vi "FestoCPX.Valve(2out2in).WithStop.vi"(4 "Delay [ms] (0)":u32, 6 "Timeout [ms] (5000)":u32=5000, 8 "error in (no error)":errorcluster, 9 "Position":T3, 10 "Valve outputs":T1[](array[typedef]), 11 "Inputs":T2[](array[typedef])) -> (0 "error out":errorcluster, 3 "Timeout?":bool)   [LabVIEW 2016]
uses:
  FestoCPX.DI.Data.States.Get.vi
  FestoCPX.DO.Data.States.Clear.vi
  FestoCPX.DI.Data.State.Get.vi
  Station/Station.ValvePosition.ctl
  FestoCPX.DI.Signal.ctl
  FestoCPX.DO.Signal.ctl
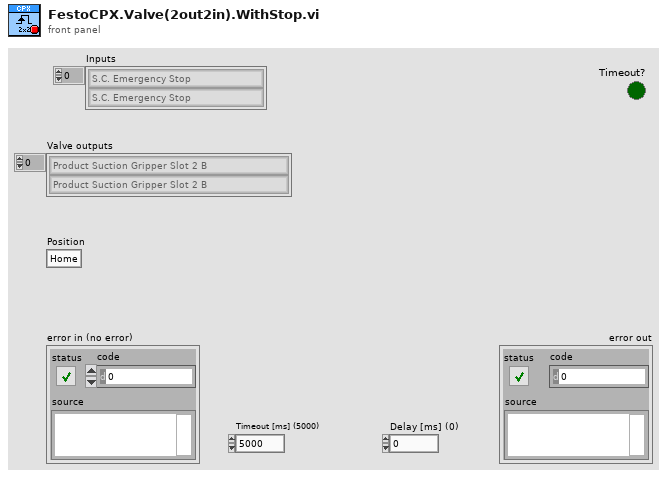
[diagram p1: front panel]
types:
  T1 = typedef "FestoCPX.DO.Signal.ctl" = enum16{"Safety Reset", "Air Main Valve", "Door Lock", "Button LED Start", "Button LED Stop", "Button LED Control", "Traffic LED Red", "Traffic LED Orange", "Traffic LED Green", "Horn", "Laser Interlock", "Laser Trigger", "Laser Fume Extractor", "Product Suction Gripper Slot 1 A", "Product Suction Gripper Slot 1 B", "Product Suction Gripper Slot 2 A", "Product Suction Gripper Slot 2 B", "Product Suction Gripper Slot 3 A", "Product Suction Gripper Slot 3 B", "Product Suction Gripper Slot 4 A", "Product Suction Gripper Slot 4 B", "Product Suction Gripper Final A", "Product Suction Gripper Final B", "Lamp", "Q1 Product Move Work", "Q1 Product Move Home", "Q2 Table Turn Work", "Q2 Table Turn Home", "Q3 Product Lift A", "Q3 Product Lift B", "Q4 Product Arm OK", "Q4 Product Arm NOK", "Q5 Product Arm Work", "Q6 Product BlowOut A", "Q6 Product BlowOut B"}
  T2 = typedef "FestoCPX.DI.Signal.ctl" = enum16{"S.C. Emergency Stop", "S.C. Side Door Close", "S.C. Front Door Close", "S.C. Front Door Secured", "Button Start", "Button Stop", "Button Control", "Product Move Home", "Product Move Work", "Table Position", "Table Lock", "Product Lift A Home", "Product Lift B Home", "Product Arm OK", "Product Arm NOK", "Product Arm Work", "Revolver ID 1", "Revolver ID 2", "Revolver ID 3", "Revolver ID 4", "Revolver ID 5", "Air Pressure Inside", "Air Pressure Inlet", "Product Slot 1 A Present", "Product Slot 1 B Present", "Product Slot 2 A Present", "Product Slot 2 B Present", "Product Slot 3 A Present", "Product Slot 3 B Present", "Product Slot 4 A Present", "Product Slot 4 B Present", "Product Final A Present", "Product Final B Present", "Product Output A Present", "Product Output B Present", "Product Container OK Present", "Product Container NOK Present", "Fork ID 1", "Fork ID 2"}
  T3 = typedef "Station.ValvePosition.ctl" = enum16{"Home", "Work"}
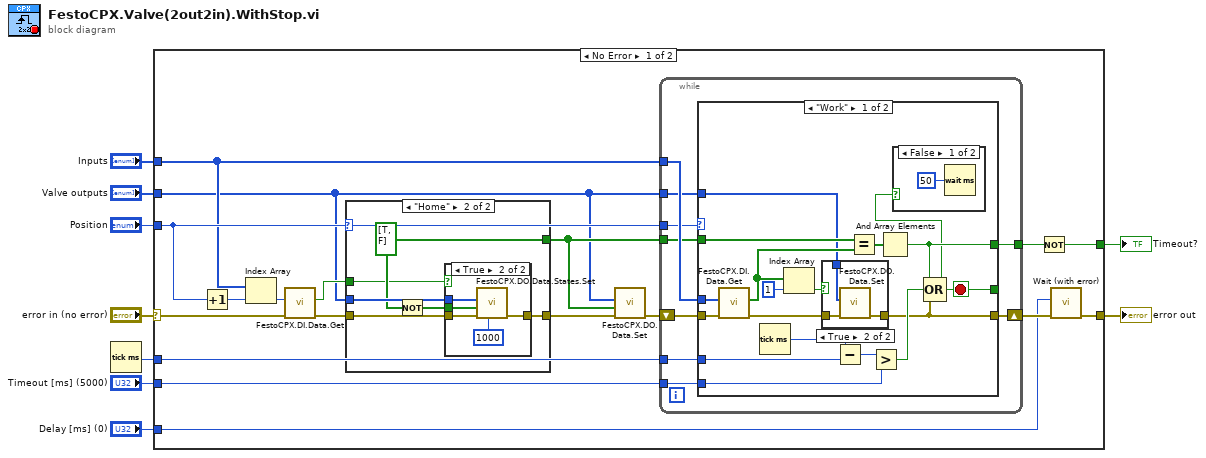
[diagram p0: block diagram]
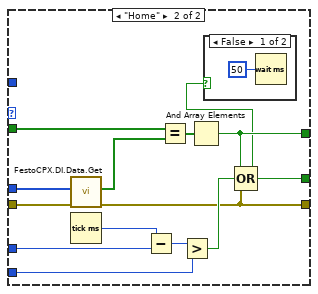
[diagram p4: hidden frame]
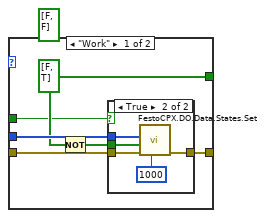
[diagram p6: hidden frame]
diagram:
  n1 = Tick Count (ms)() -> (millisecond timer value=w5:u32)
  n2 = case shown="No Error" "error in (no error)" {
    selector: "error in (no error)" -> [w16 w98]
    tunnel: "Position" -> [w14 _]
    tunnel: [w20 w98] -> w8
    tunnel: [w25 _] -> w7
    tunnel: w5 -> [w27 _]
    tunnel: "Timeout [ms] (5000)" -> [w26 _]
    tunnel: "Inputs" -> [w12 _]
    tunnel: "Valve outputs" -> [w10 _]
    tunnel: "Delay [ms] (0)" -> [w19 _]
    frame No Error {
      n3 = Increment(x=w14) -> (x+1=w17:T3)
      n4 = Index Array(array=w12, index=w17) -> (element=w18:T2)
      n5 = call-poly "FestoCPX.DI.Data.Get.vi"("error in (no error)"=w16, "CPX.DI"=w18) -> ("error out"=w15:errorcluster, "State OR"=w13:bool)  [unwired: 6 in, 2 out]
      n6 = case shown="\"Home\"" w14 {
        tunnel: [w76 w88] -> w22
        tunnel: w15 -> [w79 w91]
        tunnel: w13 -> [w74 w86]
        tunnel: [w78 w90] -> w11
        tunnel: w10 -> [w77 w89]
        frame "Work" {
          (unwired) bool[] [FALSE, FALSE]
          w76 = bool[] [FALSE, TRUE]
          n7 = Not(x=w76) -> (.not. x?=w75:bool[])
          n8 = case shown="True" w74 {
            tunnel: w79 -> [w80 w85]
            tunnel: [w80 w84] -> w78
            tunnel: w75 -> [_ w83]
            tunnel: w77 -> [_ w82]
            frame False {
            }
            frame True {
              n9 = call "FestoCPX.DO.Data.States.Set.vi"(6:u32 1000 ("Delay [ms] (0)"), "error in (no error)"=w85, "State"=w83, "CPX.DO"=w82) -> ("error out"=w84:errorcluster)  [unwired: 7 in]
            }
          }
        }
        frame "Home" {
          w88 = bool[] [TRUE, FALSE]
          n10 = Not(x=w88) -> (.not. x?=w87:bool[])
          n11 = case shown="True" w86 {
            tunnel: w91 -> [w92 w97]
            tunnel: [w92 w96] -> w90
            tunnel: w87 -> [_ w95]
            tunnel: w89 -> [_ w94]
            frame False {
            }
            frame True {
              n12 = call "FestoCPX.DO.Data.States.Set.vi"(6:u32 1000 ("Delay [ms] (0)"), "error in (no error)"=w97, "State"=w95, "CPX.DO"=w94) -> ("error out"=w96:errorcluster)  [unwired: 7 in]
            }
          }
        }
      }
      n13 = call-poly "FestoCPX.DO.Data.Set.vi"("error in (no error)"=w11, "State"=w22, "CPX.DO"=w10) -> ("error out"=w24:errorcluster)  [unwired: 8 in]
      n14 = while {
        shift-right: [w30] -> w21
        shift-left: w24 -> [w37]
        tunnel: w12 -> [w36]
        tunnel: [w32] -> w23
        tunnel: w27 -> [w35]
        tunnel: w26 -> [w34]
        tunnel: w22 -> [w33]
        tunnel: w14 -> [w29]
        tunnel: w10 -> [w28]
        stop <- w31 stop-if-true
        n15 = case shown="\"Work\"" w29 {
          tunnel: w37 -> [w54 w72]
          tunnel: w36 -> [w53 w71]
          tunnel: w35 -> [w51 w69]
          tunnel: w34 -> [w49 w67]
          tunnel: w33 -> [w48 w66]
          tunnel: [w45 w62] -> w32
          tunnel: [w44 w61] -> w31
          tunnel: [w42 w60] -> w30
          tunnel: w28 -> [w38 _]
          frame "Work" {
            n16 = call-poly "FestoCPX.DI.Data.Get.vi"("error in (no error)"=w54, "CPX.DI"=w53) -> ("error out"=w43:errorcluster, "State OR"=w41:bool[])  [unwired: 6 in, 2 out]
            n17 = Tick Count (ms)() -> (millisecond timer value=w52:u32)
            n18 = Index Array(array=w41, index=1) -> (element=w39:bool)
            n19 = case shown="True" w39 {
              tunnel: w43 -> [w55 w58]
              tunnel: [w55 w57] -> w42
              tunnel: w38 -> [_ w56]
              frame False {
              }
              frame True {
                n20 = call-poly "FestoCPX.DO.Data.Set.vi"("error in (no error)"=w58, "CPX.DO"=w56) -> ("error out"=w57:errorcluster)  [unwired: 8 in, 1 out]
              }
            }
            n21 = Subtract(x=w52, y=w51) -> (x-y=w50:u32)
            n22 = Equal?(x=w48, y=w41) -> (x = y?=w47:bool[])
            n23 = Greater?(x=w50, y=w49) -> (0:w46:bool)
            n24 = And Array Elements(Boolean array=w47) -> (logical AND=w45:bool)
            n25 = Compound Arithmetic op=OR(w45, w46, w42) -> (w44:bool)
            n26 = case shown="False" w44 {
              frame False {
                n27 = Wait (ms)(milliseconds to wait=u32 50) -> ()  [unwired: 1 out]
              }
              frame True {
              }
            }
          }
          frame "Home" {
            n28 = call-poly "FestoCPX.DI.Data.Get.vi"("error in (no error)"=w72, "CPX.DI"=w71) -> ("error out"=w60:errorcluster, "State OR"=w65:bool[])  [unwired: 6 in, 2 out]
            n29 = Tick Count (ms)() -> (millisecond timer value=w70:u32)
            n30 = Subtract(x=w70, y=w69) -> (x-y=w68:u32)
            n31 = Equal?(x=w66, y=w65) -> (x = y?=w64:bool[])
            n32 = Greater?(x=w68, y=w67) -> (0:w63:bool)
            n33 = And Array Elements(Boolean array=w64) -> (logical AND=w62:bool)
            n34 = Compound Arithmetic op=OR(w62, w63, w60) -> (w61:bool)
            n35 = case shown="False" w61 {
              frame False {
                n36 = Wait (ms)(milliseconds to wait=u32 50) -> ()  [unwired: 1 out]
              }
              frame True {
              }
            }
          }
        }
      }
      n37 = Not(x=w23) -> (.not. x?=w25:bool)
      n38 = call "Wait (with error).vi"("error in (no error)"=w21, "milliseconds to wait"=w19) -> ("error out"=w20:errorcluster)  [unwired: 8 in, 1 out]
    }
    frame Error {
    }
  }
  "error out" <- w8
  "Timeout?" <- w7
